vi "Append Table.vi"   [LabVIEW 2017, in "LabVIEW NPOI.lvlib" / "Document.lvclass"]
doc: "Appends a 2D array to the <b>Document</b> as a table. Wire data to the <B>Table</B> input to determine the polymorphic instance to use or manually select the instance."
uses:
  Document.lvclass
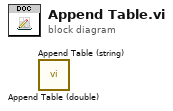
[diagram p0: block diagram]
diagram:
  n1 = call "Append Table (double).vi"() -> ()  [unwired: 14 in, 2 out]
  n2 = call "Append Table (string).vi"() -> ()  [unwired: 14 in, 2 out]
